vi "lab2ImageToChannels.vi"(2 "image data":T1) -> (3 "imgWidth":i32, 4 "imgHeight":i32, 5 "channel4":u8[](array[numeric]), 6 "redChannel":u8[](array[numeric]), 7 "greenChannel":u8[](array[numeric]), 8 "blueChannel":u8[](array[numeric]))   [LabVIEW 2016]
uses:
  <vilib>/picture/picture.llb/imagedata.ctl
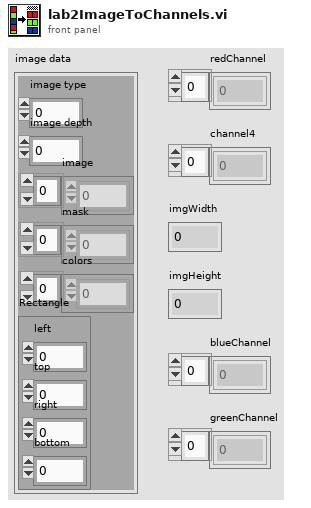
[diagram p1: front panel]
types:
  T1 = typedef "imagedata.ctl" = cluster{"image type":i32, "image depth":i32, "image":u8[], "mask":u8[], "colors":u32[], "Rectangle":cluster{"left":i16, "top":i16, "right":i16, "bottom":i16}}
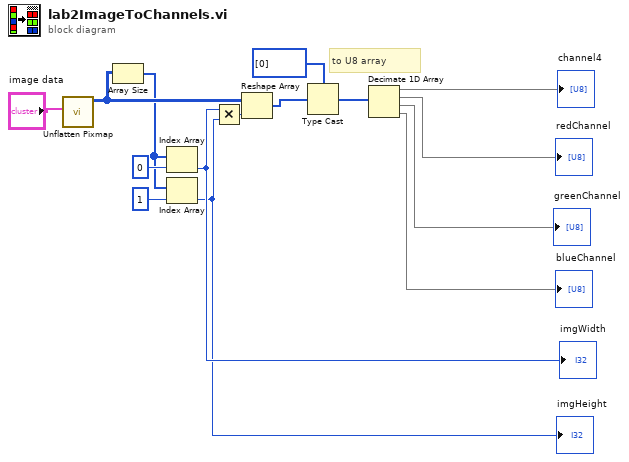
[diagram p0: block diagram]
diagram:
  # "to U8 array"
  n1 = call <vilib>:"Unflatten Pixmap.vi"("image data"="image data") -> ("24-bit pixmap"=w8:u32[][])  [unwired: 4 in, 6 out]
  n2 = Array Size(array=w8) -> (size(s)=w5:i32[])
  n3 = Index Array(array=w5, index=0) -> (element=w2:i32)
  "imgWidth" <- w2
  n4 = Index Array(array=w5, index=1) -> (element=w1:i32)
  "imgHeight" <- w1
  n5 = Multiply(x=w2, y=w1) -> (x*y=w4:i32)
  n6 = Reshape Array(w8, w4) -> (w11:u32[])
  n7 = Type Cast(type=u8[] [0], x=w11) -> (*(type *) &x=w12:u8[])
  n8 = Decimate 1D Array(w12) -> (→"channel4":u8[], →"redChannel":u8[], →"greenChannel":u8[], →"blueChannel":u8[])
